vi "Configure Jitter Measurement (N-Period).vi"(7 "Number of Periods (1)":i32=1, 8 "error in (no error)":errorcluster, 9 "N-Period Slope (0: Rising)":u16(ring) items=["Rising", "Falling"], 10 "N-Period Source (0: Channel 1)":u16(ring) items=["Channel 1", "Channel 2", "Channel 3", "Channel 4", "Math 1", "Math 2", "Math 3", "Math 4", "Reference Waveform 1", "Reference Waveform 2", "Reference Waveform 3", "Reference Waveform 4"], 11 "VISA resource name":refnum<visa-resource-name>) -> (0 "error out":errorcluster, 3 "VISA resource name out":refnum<visa-resource-name>)   [LabVIEW 2015, in "Agilent 2000 3000 X-Series.lvlib"]
doc: "Enables Jitter Analysis and configures the N-Period jitter measurement which measures the time span of N consecutive periods.\n\n<b>Note:</b>\nThis VI is specific to the 6000-X Series oscilloscopes. These features are not available on other models."
uses:
  Agilent 2000 3000 X-Series.lvlib
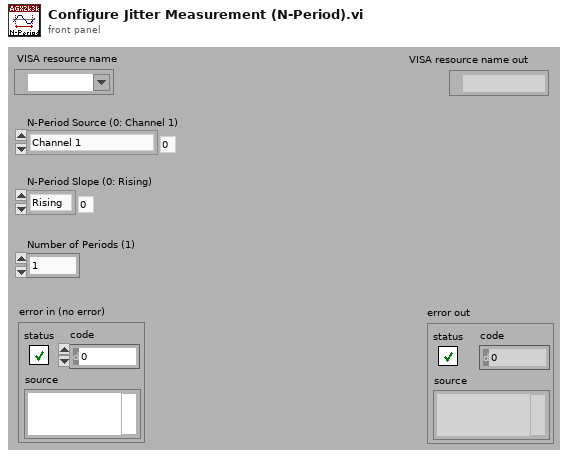
[diagram p1: front panel]
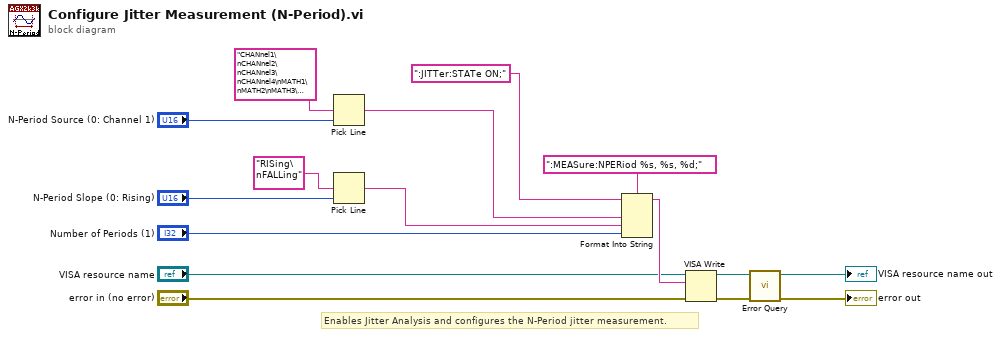
[diagram p0: block diagram]
diagram:
  # "Enables Jitter Analysis and configures the N-Period jitter measurement."
  n1 = Pick Line(multi-line string="CHANnel1\nCHANnel2\nCHANnel3\nCHANnel4\nMATH1\nMATH2\nMATH3\nMATH4\nWMEMory1\nWMEMory2\nWMEMory3\nWMEMory4", line index="N-Period Source (0: Channel 1)") -> (output string=w12:string)  [unwired: 1 in]
  n2 = Pick Line(multi-line string="RISing\nFALLing", line index="N-Period Slope (0: Rising)") -> (output string=w9:string)  [unwired: 1 in]
  n3 = Format Into String(format string=":MEASure:NPERiod %s, %s, %d;", initial string=":JITTer:STATe ON;", w12, w9, "Number of Periods (1)") -> (resulting string=w6:string)  [unwired: 1 in, 1 out]
  n4 = VISA Write(VISA resource name="VISA resource name", write buffer=w6, error in (no error)="error in (no error)") -> (VISA resource name out=w8:refnum<visa-resource-name>, error out=w7:errorcluster)  [unwired: 1 out]
  n5 = call "Error Query.vi"("error in (no error)"=w7, "VISA resource name"=w8) -> ("error out"=→"error out":errorcluster, "VISA resource name out"=→"VISA resource name out":refnum<visa-resource-name>)  [unwired: 6 in, 2 out]
